vi "Get - Scalar - Complex.vi"(7 "data type of variable":cdb, 8 "error in":errorcluster, 10 "variable name":string, 11 "pipe in":T1) -> (0 "error out":errorcluster, 2 "value":cdb format="%.2f", 3 "pipe out":T1)   [LabVIEW 2013, in "GOLPI library.lvlib"]
uses:
  GOLPI library.lvlib
  LV Process.lvlibp/Pipe Handle.ctl
  Custom Error Codes Enum Type Def.vi
  LV Process.lvlibp
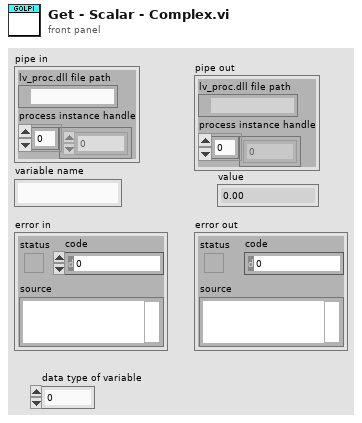
[diagram p1: front panel]
types:
  T1 = typedef "LV Process.lvlibp/Pipe Handle.ctl" = cluster{"lv_proc.dll file path":path, "process instance handle":u32[]}
  T2 = typedef "GOLPI library.lvlib/Custom Error Codes Enum Type Def.vi" = enum16{"no error", "00 working directory PAR1 missing", "01 octave binary PAR1 missing", "02 octave report error PAR1", "03 empty output last cmd PAR1", "04 missing temporary file PAR1", "10 var PAR1 not string", "11 var PAR1 not num, scal, ~compl", "12 var PAR1 not num, scal, compl", "13 var PAR1 not num, vect, ~compl", "14 var PAR1 not num, vect, compl", "15 var PAR1 not num, mat, ~compl", "16 var PAR1 not num, mat, ~compl", "99 not finished"}
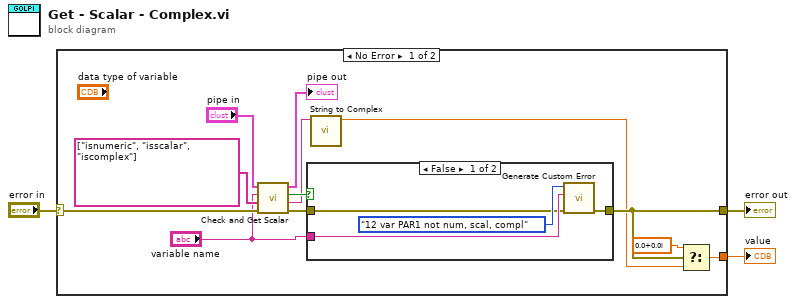
[diagram p0: block diagram]
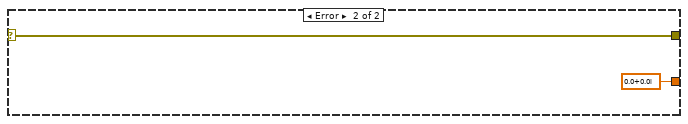
[diagram p3: hidden frame]
diagram:
  n1 = case shown="No Error" "error in" {
    selector: "error in" -> [w10 w22]
    tunnel: [w15 cdb 0.0+0.0i ("t")] -> w3
    tunnel: [w14 w22] -> w2
    frame No Error {
      n2 = call "Check and Get Scalar.vi"("error in (no error)"=w10, "test commands"=string[] ["isnumeric", "isscalar", "iscomplex"], "variable name"="variable name", "pipe in"="pipe in") -> ("error out"=w9:errorcluster, "variable"=w5:string, "all tests OK?"=w8:bool, "pipe out"=→"pipe out":T1)  [unwired: 4 in]
      n3 = case shown="False" w8 {
        tunnel: [w16 w20] -> w14
        tunnel: w9 -> [w17 w20]
        tunnel: "variable name" -> [w18 _]
        frame False {
          n4 = call "Generate Custom Error.vi"("error in"=w17, "PAR1"=w18, "Enum"=Custom_Error_Codes_Enum_Type_Def.vi."12 var PAR1 not num, scal, compl") -> ("error out"=w16:errorcluster)  [unwired: 8 in]
        }
        frame True {
        }
      }
      n5 = call "String to Complex.vi"("string"=w5) -> ("complex number"=w12:cdb)  [unwired: 10 in]
      n6 = Select(t=cdb 0.0+0.0i, s=w14, f=w12) -> (s? t:f=w15:cdb)
    }
    frame Error {
    }
  }
  "value" <- w3
  "error out" <- w2
